vi "Get output value.vi"(8 "error in (no error)":errorcluster, 11 "VISA resource name":refnum<visa-resource-name>) -> (0 "error out":errorcluster, 2 "Value":dbl, 3 "VISA resource name out":refnum<visa-resource-name>)   [LabVIEW 2012, in "Datron D4xxx.lvlib"]
doc: "This VI returns actual display value."
uses:
  Datron D4xxx.lvlib
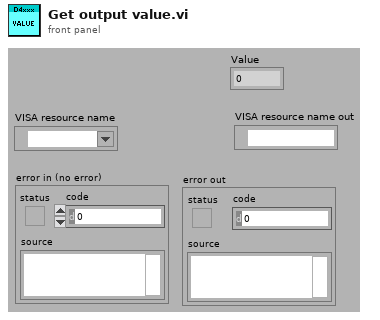
[diagram p1: front panel]
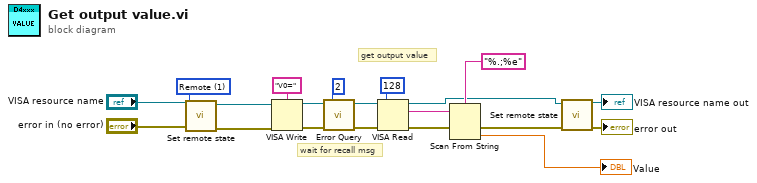
[diagram p0: block diagram]
diagram:
  w1 = u16 1 items=["Local", "Remote", "Default"] ("Remote state")
  # "wait for recall msg"
  # "get output value"
  n1 = call "Set remote state.vi"("error in"="error in (no error)", "Remote state"=w1, "VISA resource name"="VISA resource name") -> ("error out"=w4:errorcluster, "VISA resource name out"=w2:refnum<visa-resource-name>)  [unwired: 7 in]
  n2 = VISA Write(VISA resource name=w2, write buffer="V0=", error in (no error)=w4) -> (VISA resource name out=w9:refnum<visa-resource-name>, error out=w10:errorcluster)  [unwired: 1 out]
  n3 = call "Error Query.vi"("error in (no error)"=w10, "Check cycles (11)"=2, "VISA resource name"=w9) -> ("error out"=w7:errorcluster, "VISA resource name out"=w8:refnum<visa-resource-name>)  [unwired: 5 in, 2 out]
  n4 = VISA Read(VISA resource name=w8, byte count=u32 128, error in (no error)=w7) -> (VISA resource name out=w11:refnum<visa-resource-name>, read buffer=w15:string, error out=w17:errorcluster)  [unwired: 1 out]
  n5 = Scan From String(format string="%.;%e", input string=w15, error in=w17) -> (error out=w14:errorcluster, output 1=→"Value":dbl)  [unwired: 2 in, 2 out]
  n6 = call "Set remote state.vi"("error in"=w14, "VISA resource name"=w11) -> ("error out"=→"error out":errorcluster, "VISA resource name out"=→"VISA resource name out":refnum<visa-resource-name>)  [unwired: 8 in]
